vi "UI.vi"(8 "error in (no error)":errorcluster, 11 "Callback Consumer in":refnum<class "Callback Consumer.lvclass">) -> (0 "error out":errorcluster, 3 "Callback Consumer out":refnum<class "Callback Consumer.lvclass">)   [LabVIEW 2012, in "Callback Consumer.lvclass"]
uses:
  Callback Consumer.lvclass
panel:
  out "Numeric":dbl
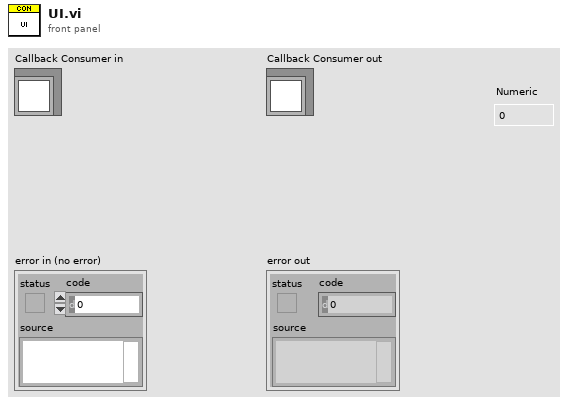
[diagram p1: front panel]
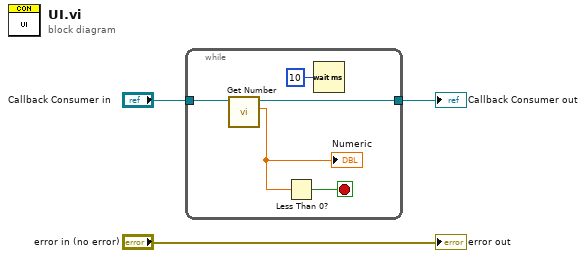
[diagram p0: block diagram]
diagram:
  n1 = while {
    tunnel: "Callback Consumer in" -> [w8]
    tunnel: [w7] -> w1
    stop <- w5 stop-if-true
    n2 = call "Get Number.vi"("Callback Consumer in"=w8) -> ("Numeric"=w6:dbl, "Callback Consumer out"=w7:refnum<class "Callback Consumer.lvclass">)  [unwired: 8 in, 1 out]
    "Numeric" <- w6
    n3 = Less Than 0?(x=w6) -> (x < 0?=w5:bool)
    n4 = Wait (ms)(milliseconds to wait=u32 10) -> ()  [unwired: 1 out]
  }
  "Callback Consumer out" <- w1
  "error out" <- "error in (no error)"
